vi "Run 1.vi"   [LabVIEW 2016]
types:
  T1 = typedef "LVHSConnector.ctl" = refnum<class "BrickReference.lvclass">
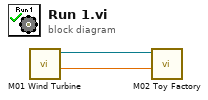
[diagram p0: block diagram]
diagram:
  n1 = call "M01 Wind Turbine.vi"() -> ("Angle out"=w1:sgl, "EV3 out"=w2:T1)  [unwired: 10 in]
  n2 = call "M02 Toy Factory.vi"("Angle in"=w1, "EV3 in"=w2) -> ()  [unwired: 9 in, 1 out]
